vi "IMU code drive straight.vi"() -> ()   [LabVIEW 2017]
uses:
  <vilib>/Rock Robotics/WPI/Utilities/WPI_GetSetVariantRefNum.vi
  <vilib>/addons/control/pid/pid.llb/PID (DBL).vi
  <vilib>/Rock Robotics/WPI/RobotDrive/WPI_RobotDriveArcadeDrive_Standard(NoSaturation).vi
  <vilib>/Rock Robotics/Network Tables/NT Write Numeric Array.vi
  <vilib>/Rock Robotics/Network Tables/NT Read Number.vi
  <vilib>/Rock Robotics/WPI/ThirdParty/Sensors/ADIS16448 IMU/ADIS16448_IMU.lvlib
  <vilib>/addons/control/pid/NI_PID_pid.lvlib
panel:
  out "Z Angle":dbl
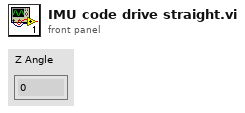
[diagram p1: front panel]
types:
  T1 = cluster{"proportional gain (Kc)":dbl, "integral time (Ti, min)":dbl, "derivative time (Td, min)":dbl}
  T2 = typedef "ADIS16448_IMU.lvlib/ADI_IMU_ADIS16448_IMUDevRef.ctl" = cluster{"DevStatus":errorcluster, "Handle":i32, "SPI Bus":T3, "Device Found":bool, "Device Ready":bool, "Yaw Axis":enum16{"X", "Y", "Z"}, "AHRS Algorithm":enum16{"Complementary", "Madgwick"}, "Serial":u16, "Lot ID 2":u16, "Lot ID 1":u16, "Bytes Per Sample":u16, "Calibrate On Open?":bool}
  T3 = typedef "spi_bus.ctl" = enum16{"SPI On-Board, CS0", "SPI On-Board, CS1", "SPI On-Board, CS2", "SPI On-Board, CS3", "SPI MXP", "Invalid"}
  T4 = cluster{"X Angle":dbl, "Y Angle":dbl, "Z Angle":dbl}
  T5 = typedef "WPI_RobotDriveDevRef.ctl" = cluster{"DevStatus":errorcluster, "Motors[]":T6[], "Square Inputs":bool, "Max Output":dbl}
  T6 = typedef "WPI_MotorControlDeviceRef.ctl" = cluster{"DeviceStatus":errorcluster, "Type":T7, "PWM":cluster{"PWM Channel":T8, "DeadBand":T9}, "CAN":cluster{"Device Number":u8, "SetOutput VI Ref":variant, "GetOutput VI Ref":variant, "Enable VI Ref":variant, "Disable VI Ref":variant, "Data":variant}, "Invert":bool, "DIO PWM":cluster{"PWM \"Enable\" Channel":T8, "DIOChannel":T10, "PWM Rate":dbl}}
  T7 = typedef "WPI_MotorControlType.ctl" = enum16{"PWM", "CAN", "DIO PWM"}
  T8 = typedef "FPGA_DIOPWMChannel.ctl" = enum8{"PWM 0", "PWM 1", "PWM 2", "PWM 3", "PWM 4", "PWM 5", "PWM 6", "PWM 7", "PWM 8", "PWM 9", "PWM MXP 0", "PWM MXP 1", "PWM MXP 2", "PWM MXP 3", "PWM MXP 4", "PWM MXP 5", "PWM MXP 6", "PWM MXP 7", "PWM MXP 8", "PWM MXP 9", "Invalid"}
  T9 = typedef "WPI_PWMDeadband.ctl" = cluster{"Name":string, "maxPositivePwm":i32, "minPositivePwm":i32, "centerPwm":i32, "maxNegativePwm":i32, "minNegativePwm":i32, "angularRange":u16}
  T10 = typedef "FPGA_DIOChannel.ctl" = enum8{"DIO 0", "DIO 1", "DIO 2", "DIO 3", "DIO 4", "DIO 5", "DIO 6", "DIO 7", "DIO 8", "DIO 9", "DIO MXP 0", "DIO MXP 1", "DIO MXP 2", "DIO MXP 3", "DIO MXP 4", "DIO MXP 5", "DIO MXP 6", "DIO MXP 7", "DIO MXP 8", "DIO MXP 9", "DIO MXP 10", "DIO MXP 11", "DIO MXP 12", "DIO MXP 13", "DIO MXP 14", "DIO MXP 15", "SPI Port CS1", "SPI Port CS2", "SPI Port CS3", "SPI Port MISO", "SPI Port MOSI", "Invalid"}
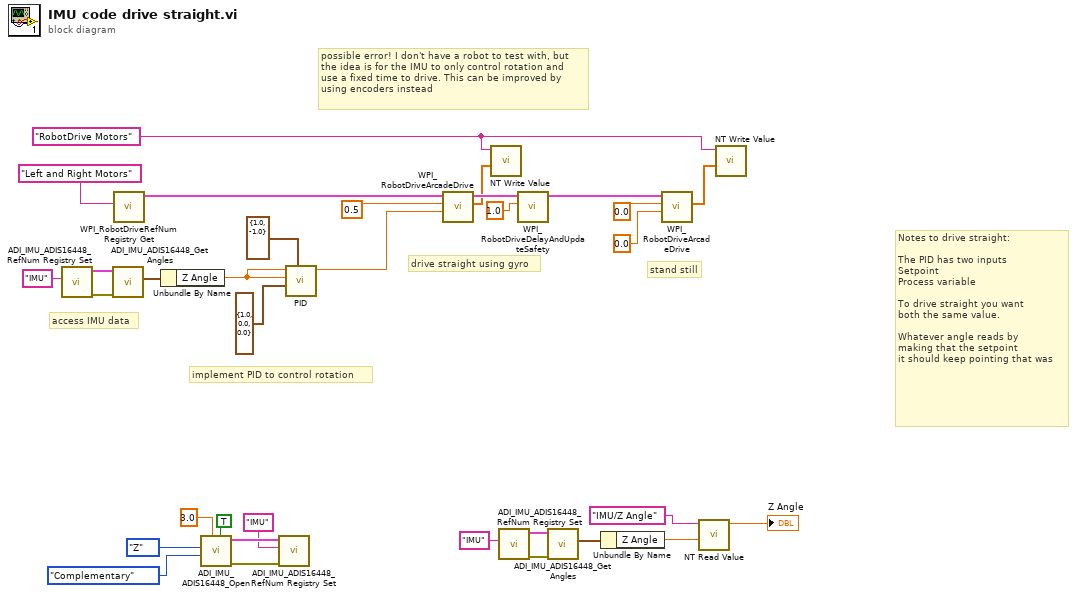
[diagram p0: block diagram]
diagram:
  w25 = "RobotDrive Motors" ("Name")
  # "Notes to drive straight:\n\nThe PID has two inputs\nSetpoint\nProcess variable\n\nTo drive straight you want\nboth the same value.\n\nWhatever angle reads by \nmaking that the setpoint\nit should keep pointing that was"
  # "possible error! I don't have a robot to test with, but\nthe idea is for the IMU to only control rotation and\nuse a fixed time to drive. This can be improved by \nusing encoders instead"
  # "implement PID to control rotation"
  # "access IMU data"
  # "stand still"
  # "drive straight using gyro"
  n1 = call <vilib>:"ADI_IMU_ADIS16448_RefNum Registry Set.vi"("refnum name"="IMU") -> ("error out"=w21:errorcluster, "ADI IMU DevRef"=w20:T2)  [unwired: 9 in]
  n2 = call <vilib>:"ADI_IMU_ADIS16448_Get Angles.vi"("error in"=w21, "ADI IMU DevRef"=w20) -> ("IMU Angles Out"=w19:T4)  [unwired: 6 in, 3 out]
  n3 = call <vilib>:"WPI_RobotDriveRefNum Registry Get.vi"("refnum name"="Left and Right Motors") -> ("RobotDriveDevRef"=w33:T5)  [unwired: 1 in, 9 out]
  n4 = Unbundle By Name(w19) -> ("Z Angle"=w18:dbl)
  n5 = call <vilib>:"ADI_IMU_ADIS16448_Open.vi"("Calibrate On Open"=TRUE, "Calibration Time (s)"=3.0, "AHRS Algorithm"=enum16{"Complementary", "Madgwick"}."Complementary", "Yaw Axis"=enum16{"X", "Y", "Z"}."Z") -> ("error out"=w10:errorcluster, "ADI IMU DevRef Out"=w9:T2)  [unwired: 5 in, 1 out]
  n6 = call <vilib>:"ADI_IMU_ADIS16448_RefNum Registry Set.vi"("error in (no error)"=w10, "refnum name"="IMU", "ADI IMU DevRef"=w9) -> ()  [unwired: 7 in, 2 out]
  n7 = call-poly <vilib>:"PID.vi"("output range"=cluster{"output high":dbl, "output low":dbl} {"output high"=1.0, "output low"=-1.0}, "PID gains"=T1 {"proportional gain (Kc)"=1.0, "integral time (Ti, min)"=0.0, "derivative time (Td, min)"=0.0}, "process variable"=w18, "setpoint"=w18) -> ("output"=w15:dbl)  [unwired: 6 in, 1 out]
  n8 = call-poly <vilib>:"WPI_RobotDriveArcadeDrive.vi"("Y axis value"=w15, "X axis value"=0.5, "RobotDriveDevRef"=w33) -> ("Motor Values"=w24:dbl[], "RobotDriveDevRef"=w30:T5)  [unwired: 1 in, 6 out]
  n9 = call-poly <vilib>:"NT Write Value.vi"("Numeric Array"=w24, "Name"=w25) -> ()  [unwired: 9 in, 1 out]
  n10 = call <vilib>:"ADI_IMU_ADIS16448_RefNum Registry Set.vi"("refnum name"="IMU") -> ("error out"=w6:errorcluster, "ADI IMU DevRef"=w5:T2)  [unwired: 9 in]
  n11 = call <vilib>:"WPI_RobotDriveDelayAndUpdateSafety.vi"("Delay (s)"=1.0, "RobotDriveDevRef"=w30) -> ("RobotDriveDevRef 2"=w23:T5)  [unwired: 8 in, 1 out]
  n12 = call <vilib>:"ADI_IMU_ADIS16448_Get Angles.vi"("error in"=w6, "ADI IMU DevRef"=w5) -> ("IMU Angles Out"=w4:T4)  [unwired: 6 in, 3 out]
  n13 = Unbundle By Name(w4) -> ("Z Angle"=w3:dbl)
  n14 = call-poly <vilib>:"WPI_RobotDriveArcadeDrive.vi"("Y axis value"=0.0 ("X axis value"), "X axis value"=0.0, "RobotDriveDevRef"=w23) -> ("Motor Values"=w26:dbl[])  [unwired: 1 in, 7 out]
  n15 = call-poly <vilib>:"NT Read Value.vi"("Default Value"=w3, "Name"="IMU/Z Angle") -> ("Numeric"=→"Z Angle":dbl)  [unwired: 8 in, 1 out]
  n16 = call-poly <vilib>:"NT Write Value.vi"("Numeric Array"=w26, "Name"=w25) -> ()  [unwired: 9 in, 1 out]
